vi "reset gyro.vi"() -> ()   [LabVIEW 2018]
panel:
  in  "Reset Gyro":bool
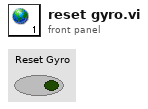
[diagram p1: front panel]
diagram:
